vi "GetWidthAndHeight.vi"(0 "Camera Cluster":T2) -> (1 "Width":u32, 2 "Height":u32)   [LabVIEW 2010]
uses:
  <vilib>/userDefined/High Color/IMAQdx.ctl
  Program Files (x86)/National Instruments/LabVIEW 2010/resource/objmgr/imaqdx.rc
  Image-Stack-Compressor/Stack Reader Wrapper/labview vis/StackReaderWrapper.lvlib
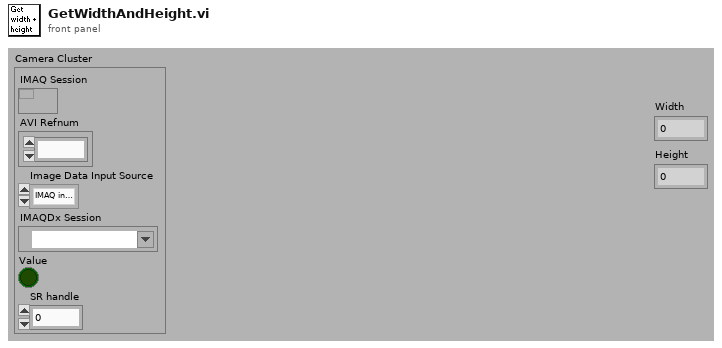
[diagram p1: front panel]
types:
  T1 = typedef "IMAQdx.ctl" = refnum<k21>
  T2 = cluster{"IMAQ Session":refnum<k11>, "AVI Refnum":refnum<k1>, "Image Data Input Source":enum32{"IMAQ interface", "IMAQdx interface", "AVI file", "MMF File"}, "IMAQDx Session":T1, "Value":bool, "SR handle":u32}
  T3 = enum32{"IMAQ interface", "IMAQdx interface", "AVI file", "MMF File"}
  T4 = cluster{"width":u32, "height":u32, "framesPerSecond":u32, "compressionFilter":string, "hasData":bool}
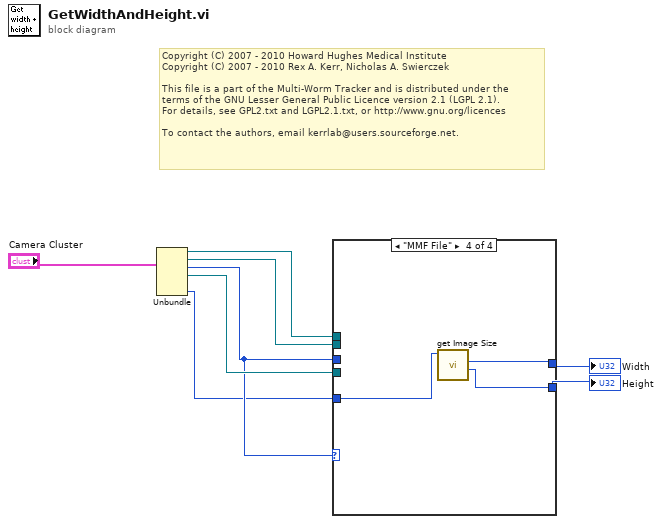
[diagram p0: block diagram]
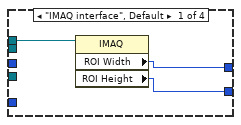
[diagram p2: hidden frame]
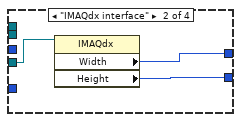
[diagram p3: hidden frame]
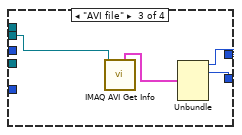
[diagram p4: hidden frame]
diagram:
  # "Copyright (C) 2007 - 2010 Howard Hughes Medical Institute\nCopyright (C) 2007 - 2010 Rex A. Kerr, Nicholas A. Swierczek\n \nThis file is a part of the Multi-Worm Tracker and is distributed under the\nterms of the GNU Lesser General Public Licence version 2.1 (LGPL 2.1).\nFor details, see GPL2.txt and LGPL2.1.txt, or http://www.gnu.org/licences\n \nTo contact the authors, email kerrlab@users.sourceforge.net."
  n1 = Unbundle("Camera Cluster") -> ("IMAQ Session"=w8:refnum<k11>, "AVI Refnum"=w4:refnum<k1>, "Image Data Input Source"=w3:T3, "IMAQDx Session"=w5:T1, "SR handle"=w1:u32)  [unwired: 1 out]
  n2 = case shown="\"MMF File\"" w3 {
    tunnel: w5 -> [_ w12 _ _]
    tunnel: w8 -> [w11 _ _ _]
    tunnel: [w10 w14 w17 w20] -> w7
    tunnel: [w9 w13 w16 w19] -> w6
    tunnel: w3 -> [_ _ _ _]
    tunnel: w4 -> [_ _ w15 _]
    tunnel: w1 -> [_ _ _ w21]
    frame "IMAQ interface", Default {
      n3 = property class="IMAQ"(reference=w11) -> ("ROI Width"=w10:u32, "ROI Height"=w9:u32)  [unwired: 1 in, 2 out]
    }
    frame "IMAQdx interface" {
      n4 = property class="IMAQdx"(reference=w12) -> ("Width"=w14:u32, "Height"=w13:u32)  [unwired: 1 in, 2 out]
    }
    frame "AVI file" {
      n5 = call "IMAQ AVI Get Info"("Avi Refnum"=w15) -> ("Frame Data"=w18:T4)  [unwired: 6 in, 4 out]
      n6 = Unbundle(w18) -> ("width"=w17:u32, "height"=w16:u32)  [unwired: 3 out]
    }
    frame "MMF File" {
      n7 = call "get Image Size.vi"("SR"=w21) -> ("height"=w19:i32, "width"=w20:i32)  [unwired: 7 in, 2 out]
    }
  }
  "Width" <- w7
  "Height" <- w6
